vi "WIPE.vi"(8 "error in (no error)":errorcluster, 11 "connection ID":refnum<k16>) -> (0 "error out":errorcluster, 2 "data out":string, 3 "connection ID out":refnum<k16>)   [LabVIEW 2018]
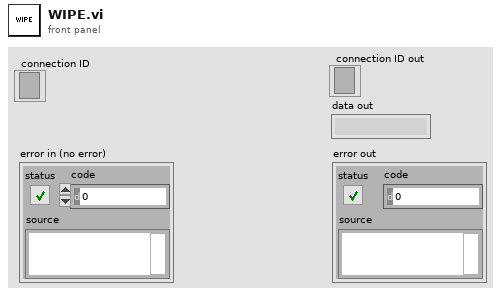
[diagram p1: front panel]
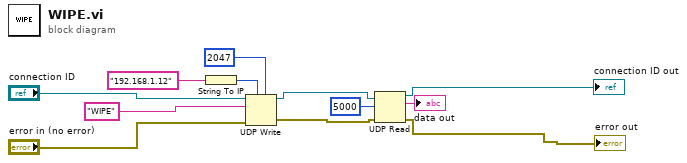
[diagram p0: block diagram]
diagram:
  n1 = String To IP(1:"192.168.1.12" ("name")) -> (0:w11:u32)
  n2 = UDP Write(address=w11, port or service name=u16 2047, connection ID="connection ID", data in="WIPE", 8:"error in (no error)") -> (error out=w5:errorcluster, 3:w6:refnum<k16>)  [unwired: 1 in]
  n3 = UDP Read(connection ID=w6, max size (548)=5000 ("timeout ms (25000)"), 8:w5) -> (data out=→"data out":string, error out=→"error out":errorcluster, 3:→"connection ID out":refnum<k16>)  [unwired: 1 in, 2 out]
